vi "Module Init.vi"(8 "error in (no error)":errorcluster, 11 "GenericGuiAI in":refnum<class "GenericGuiAI.lvclass">) -> (0 "error out":errorcluster, 3 "GenericGuiAI out":refnum<class "GenericGuiAI.lvclass">)   [LabVIEW 2020, in "VolatusDAQGenericGUI.lvlib" / "GenericGuiAI.lvclass"]
uses:
  GenericGuiAI.lvclass
  C:/dev/lv20CE/relink/lv-volatus/Volatus/Module/Module.lvclass
  VolatusConfig/Meta Type.ctl
  VolatusConfig/Meta Name.ctl
  Volatus/Module/Module.lvclass/Module.ctl
  VolatusConfig/VolatusConfigElement/VolatusConfigElement.lvclass/VolatusConfigElement.ctl
  GenericGuiAI.lvclass/GenericGuiAI.ctl
  VolatusConfig/VolatusConfigElement/Element.vi
  lv-cdm/CDM-Config/Config Lookup/Match Meta.vi
  lv-cdm/CDM-Config/Config Element/Owner.vi
  lv-cdm/CDM-Config/Config Manager/Lookup Descendant.vi
  VolatusConfig/Group/Group.lvclass
  lv-cdm/CDM-Config/Config Filter/Config Lookup.lvclass
  Volatus/Module/Module.lvclass
  VolatusConfig/VolatusConfigElement/VolatusConfigElement.lvclass
  VolatusConfig/VolatusConfig.lvlib
  lv-cdm/CDM-Config/Config Element/Config Element.lvclass
  VolatusConfig/Task/Task.lvclass
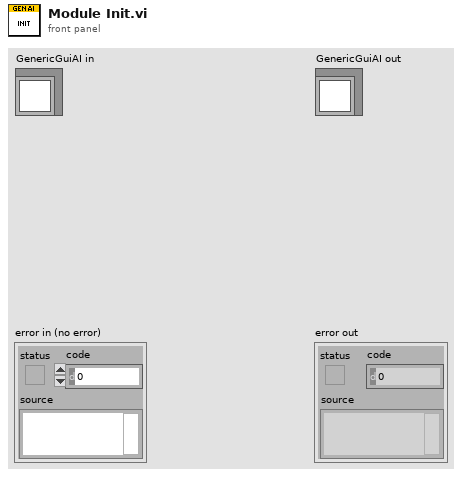
[diagram p1: front panel]
types:
  T1 = typedef "VolatusConfig.lvlib/Meta Name.ctl" = enum16{"VL_Type", "VL_Node_IP", "VL_Node_Type", "VL_Task_Type", "VL_Group_Type", "VL_Channel_Type", "VL_Channel_DataType", "VL_Config_Version", "VL_Overlay_Type"}
  T2 = typedef "VolatusConfig.lvlib/Meta Type.ctl" = enum16{"UNKNOWN", "VL_System", "VL_Cluster", "VL_Node", "VL_Task", "VL_Group", "VL_Channel", "VL_Task_List", "VL_Scaling", "VL_Sensor", "VL_Sensor_List", "VL_Scale"}
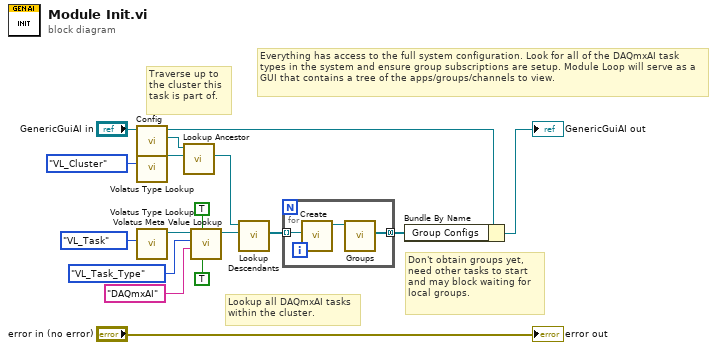
[diagram p0: block diagram]
diagram:
  # "Don't obtain groups yet, need other tasks to start and may block waiting for local groups."
  # "Lookup all DAQmxAI tasks within the cluster."
  # "Traverse up to the cluster this task is part of."
  # "Everything has access to the full system configuration. Look for all of the DAQmxAI task types in the system and ensure group subscriptions are setup. Module Loop will serve as a GUI that contains a tree of the apps/groups/channels to view."
  n1 = call "Config.vi"("Module in"="GenericGuiAI in") -> ("Config"=w16:refnum<class "VolatusConfigElement.lvclass">, "Module out"=w4:refnum<class "GenericGuiAI.lvclass">)  [unwired: 9 in]
  n2 = call "Volatus Type Lookup.vi"("Meta Type"=Meta_Type."VL_Cluster") -> ("Config Lookup out"=w15:refnum<class "Config Lookup.lvclass">)  [unwired: 9 in, 1 out]
  n3 = call "Volatus Type Lookup.vi"("Meta Type"=Meta_Type."VL_Task") -> ("Config Lookup out"=w11:refnum<class "Config Lookup.lvclass">)  [unwired: 9 in, 1 out]
  n4 = call "Lookup Ancestor.vi"("Lookup"=w15, "VolatusConfigElement in"=w16) -> ("Ancestor"=w13:refnum<class "Config Element.lvclass">)  [unwired: 7 in, 2 out]
  n5 = call "Volatus Meta Value Lookup.vi"("Exact Value (F)"=TRUE, "Don't Recurse Past Match (F)"=TRUE, "Value"="DAQmxAI", "Meta Name"=Meta_Name."VL_Task_Type", "Config Lookup (New)"=w11) -> ("Config Lookup out"=w7:refnum<class "Config Lookup.lvclass">)  [unwired: 5 in, 1 out]
  n6 = call "Lookup Descendants.vi"("Lookup"=w7, "Config Element in"=w13) -> ("Descendants"=w6:refnum<class "Config Element.lvclass">[])  [unwired: 7 in, 2 out]
  n7 = for {
    tunnel: w6 -> [w20] mode=indexing
    tunnel: [w18] -> w3 mode=concatenating
    n8 = call "Create.vi"("Element"=w20) -> ("Task out"=w19:refnum<class "Task.lvclass">)  [unwired: 9 in, 1 out]
    n9 = call "Groups.vi"("Task in"=w19) -> ("Groups"=w18:refnum<class "Group.lvclass">[])  [unwired: 8 in, 2 out]
  }
  n10 = Bundle By Name(cluster=w4, "Group Configs"=w3) -> (→"GenericGuiAI out":refnum<class "GenericGuiAI.lvclass">)
  "error out" <- "error in (no error)"
